vi "Read.vi"   [LabVIEW 2011, in "LVH-Adept.lvlib"]
doc: "Read data from a Digilent FPGA board that has been configured for use with the Adept interface."
uses:
  <vilib>/LabVIEW Hacker/Adept/LVH-Adept.lvlib
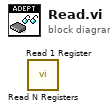
[diagram p0: block diagram]
diagram:
  n1 = call "Read N Registers.vi"() -> ()  [unwired: 9 in, 3 out]
  n2 = call "Read 1 Register.vi"() -> ()  [unwired: 9 in, 3 out]
